vi "Modify Forecast Data.vi"(8 "error in":errorcluster, 9 "dt (sec)":dbl, 10 "t0 (sec)":dbl, 11 "array":dbl[](array[numeric])) -> (0 "dup error out":errorcluster, 3 "Data":dbl[](array[numeric]))   [LabVIEW 2018, in "Generic Optimization Actor.lvlib" / "Generic Optimization.lvclass"]
uses:
  Generic Optimization.lvclass
  <vilib>/gmath/NI_Gmath.lvlib
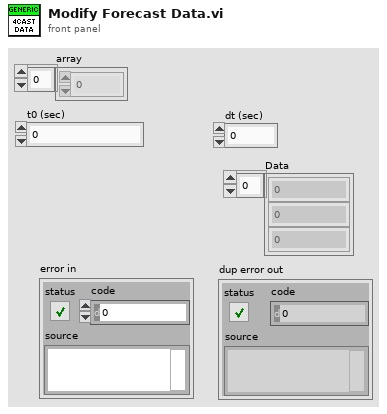
[diagram p1: front panel]
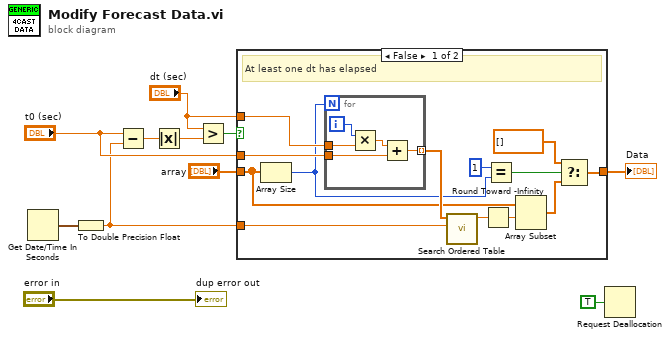
[diagram p0: block diagram]
diagram:
  n1 = Get Date/Time In Seconds() -> (seconds since 1Jan1904=w10:timestamp)
  n2 = To Double Precision Float(number=w10) -> (double precision float=w3:dbl)
  n3 = Subtract(x="t0 (sec)", y=w3) -> (x-y=w9:dbl)
  n4 = Absolute Value(x=w9) -> (abs(x)=w8:dbl)
  n5 = Greater?(x="dt (sec)", y=w8) -> (0:w7:bool)
  n6 = case shown="False" w7 {
    tunnel: "array" -> [w18 w30]
    tunnel: "t0 (sec)" -> [w24 _]
    tunnel: "dt (sec)" -> [w23 _]
    tunnel: w3 -> [w21 _]
    tunnel: [w13 w30] -> w2
    frame False {
      # "At least one dt has elapsed"
      n7 = Array Size(array=w18) -> (size(s)=w17:i32)
      n8 = for {
        N: w17 -> [_]
        tunnel: w24 -> [w29]
        tunnel: w23 -> [w26]
        tunnel: [w28] -> w22 mode=indexing
        i -> [w27]
        n9 = Multiply(x=w27, y=w26) -> (x*y=w25:dbl)
        n10 = Add(x=w25, y=w29) -> (x+y=w28:dbl)
      }
      n11 = call <vilib>:"Search Ordered Table.vi"("x value"=w21, "ordered x array"=w22) -> ("fractional index"=w20:dbl)  [unwired: 9 in]
      n12 = Round Toward -Infinity(1:w20) -> (0:w19:dbl)
      n13 = Equal?(x=1, y=w17) -> (x = y?=w15:bool)
      n14 = Array Subset(array=w18, index=w19) -> (w14:dbl[])  [unwired: 1 in]
      n15 = Select(t=dbl[] [], s=w15, f=w14) -> (s? t:f=w13:dbl[])
    }
    frame True {
      # "dt has not yet elapsed. pass current array through"
    }
  }
  "Data" <- w2
  n16 = Request Deallocation(TRUE ("flag")) -> ()
  "dup error out" <- "error in"
